vi "State_Connect.vi"(8 "error in (no error)":errorcluster, 9 "Parameter":variant, 10 "Command":string, 11 "MB Slave in":refnum<class "MB Slave Simulator Base.lvclass">) -> (0 "error out":errorcluster, 2 "Debug Message":string, 3 "MB Slave out":refnum<class "MB Slave Simulator Base.lvclass">)   [LabVIEW 2021, in "MB Slave Simulator Base.lvclass"]
uses:
  MB Slave Simulator Base.lvclass
  MB Slave Simulator Base.lvclass/MB Slave Simulator Base.ctl
  Accessors/Write Initialized.vi
  <userlib>/S2 Labs/Module Framework/Modules/Modbus/Modbus Slave Base/Modbus Slave Base.lvclass
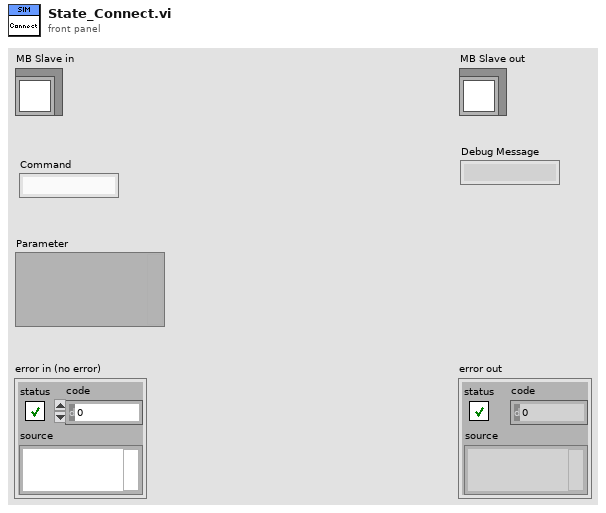
[diagram p1: front panel]
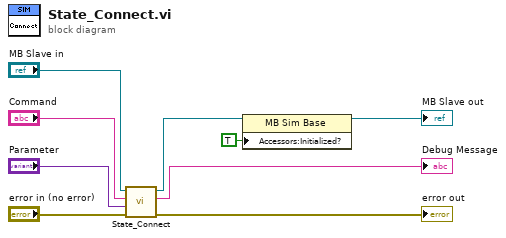
[diagram p0: block diagram]
diagram:
  n1 = call-parent "State_Connect.vi"("error in (no error)"="error in (no error)", "Parameter"="Parameter", "Command"="Command", "MB Slave in"="MB Slave in") -> ("error out"=→"error out":errorcluster, "Debug Message"=→"Debug Message":string, "MB Slave out"=w2:refnum<class "MB Slave Simulator Base.lvclass">)  [unwired: 5 in]
  n2 = property class="MB Sim Base"(reference=w2, "Accessors:Initialized?"=TRUE ("Initialized?")) -> (reference out=→"MB Slave out":refnum<class "MB Slave Simulator Base.lvclass">)  [unwired: 1 in, 1 out]
